vi "analizor.vi"() -> ()   [LabVIEW 2011]
uses:
  <vilib>/Analysis/4window.llb/windowTd.ctl
  <vilib>/Waveform/WDTOps.llb/WDT Append Waveforms DBL.vi
  <vilib>/measure/maspectr.llb/FFT Power Spectrum and PSD for 1 Chan.vi
  <vilib>/measure/NI_MABase.lvlib
  <vilib>/measure/NI_MAPro.lvlib
  <vilib>/Analysis/NI_AALPro.lvlib
panel:
  in  "path":path
  in  "dB On (F)":bool
  in  "window":T1=1 items=["Rectangle"=0, "Hanning"=1, "Hamming"=2, "Blackman-Harris"=3, "Exact Blackman"=4, "Blackman"=5, "Flat Top"=6, "4 Term B-Harris "=7, "7 Term B-Harris"=8, "Low Sidelobe"=9, "Blackman Nuttall"=11, "Triangle"=30, "Bartlett-Hanning"=31, "Bohman"=32, "Parzen"=33, "Welch"=34, "Kaiser"=60, "Dolph-Chebyshev"=61, "Gaussian"=62]
  in  "Amplitude":dbl
  in  "Frequency (Hz)":dbl(knob) scale=0.0..500.0
  out "Waveform Graph":cluster{"f0":dbl, "df":dbl, "magnitude":dbl[]}(graph)
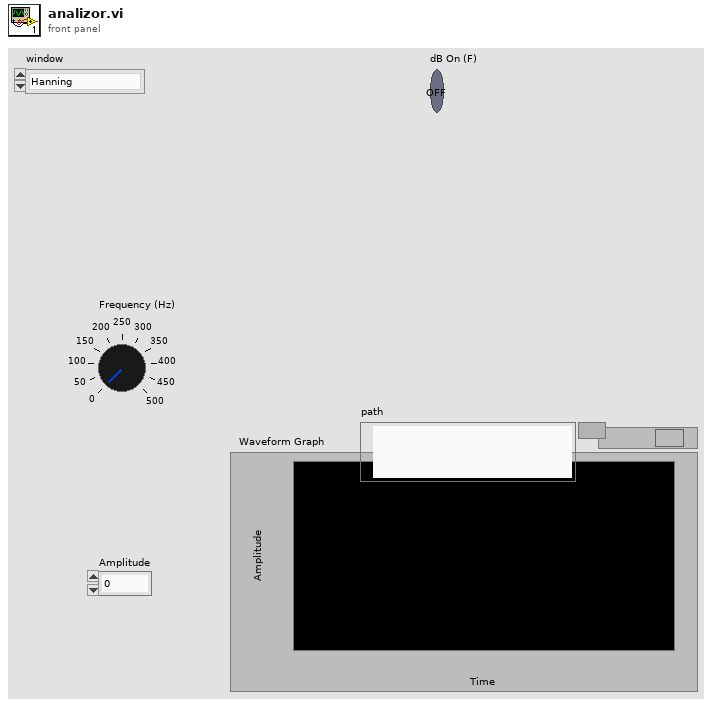
[diagram p1: front panel]
types:
  T1 = typedef "NI_AALPro.lvlib/windowTd.ctl" = u32
  T2 = cluster{"averaging mode":enum16{"No averaging", "Vector averaging", "RMS averaging", "Peak hold"}, "weighting mode":enum16{"Linear", "Exponential"}, "number of averages":u32}
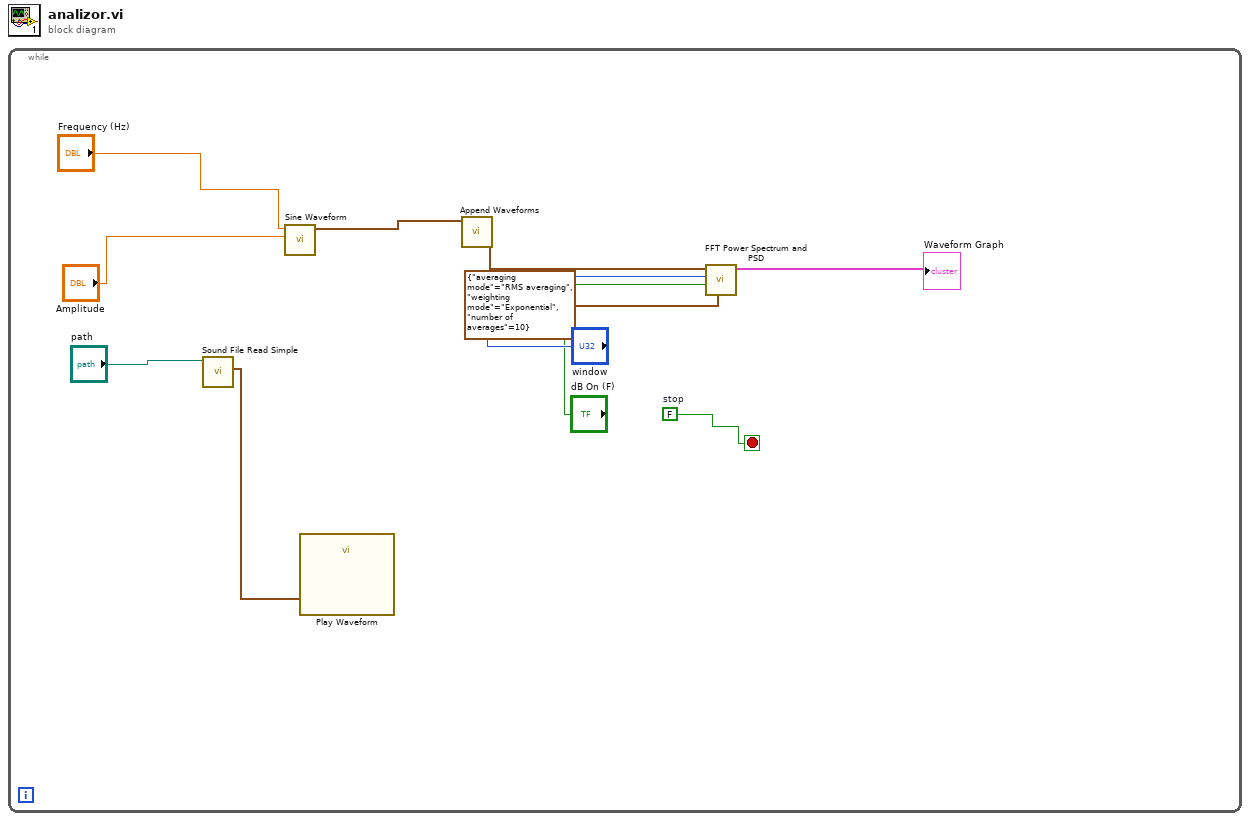
[diagram p0: block diagram]
diagram:
  n1 = while {
    stop <- w6 stop-if-true
    w6 = FALSE  # stop
    n2 = call <vilib>:"Sound File Read Simple.vi"("path"="path") -> ("data"=w2:waveform(dbl)[])  [unwired: 7 in, 3 out]
    n3 = call <vilib>:"Sine Waveform.vi"("amplitude"="Amplitude", "frequency"="Frequency (Hz)") -> ("signal out"=w9:waveform(dbl))  [unwired: 8 in, 1 out]
    n4 = call "Play Waveform"("Data"=w2) -> ()  [unwired: 18 in, 1 out]
    n5 = call-poly <vilib>:"Append Waveforms.vi"("waveform A"=w9) -> ("waveform out"=w8:waveform(dbl))  [unwired: 9 in, 1 out]
    n6 = call-poly <vilib>:"FFT Power Spectrum and PSD.vi"("averaging parameters"=T2 {"averaging mode"=enum."RMS averaging", "weighting mode"=enum."Exponential", "number of averages"=10}, "dB On (F)"="dB On (F)", "window"="window", "time signal"=w8) -> ("Power Spectrum / PSD"=→"Waveform Graph":cluster{"f0":dbl, "df":dbl, "magnitude":dbl[]})  [unwired: 4 in, 3 out]
  }
